vi "Periodic Tasks.vi"(8 "error in":errorcluster) -> ()   [LabVIEW 2013]
doc: "This VI runs in parallel to other tasks. It can contain as many user-defined periodic loops as you need. These can carry out PID or other sorts of timed response."
uses:
  <vilib>/Rock Robotics/SystemInterfaces/Utilities/FPGA_UtilitiesLED Source.ctl
  <vilib>/Rock Robotics/SystemInterfaces/Utilities/FPGA_UtilitiesLED State.ctl
  Robot Global Data.vi
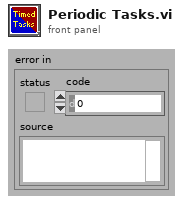
[diagram p1: front panel]
types:
  T1 = typedef "FPGA_UtilitiesLED State.ctl" = enum16{"Off", "On", "Toggle"}
  T2 = typedef "FPGA_UtilitiesLED Source.ctl" = enum16{"User LED", "FPGA LED"}
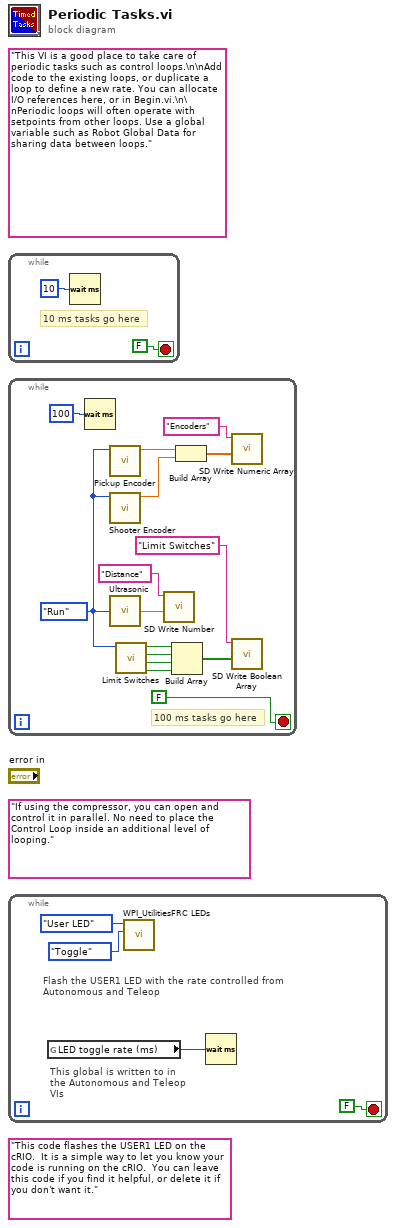
[diagram p0: block diagram]
diagram:
  (unwired) "If using the compressor, you can open and control it in parallel. No need to place the Control Loop inside an additional level of looping."
  (unwired) "This code flashes the USER1 LED on the cRIO.  It is a simple way to let you know your code is running on the cRIO.  You can leave this code if you find it helpful, or delete it if you don't want it."
  (unwired) "This VI is a good place to take care of periodic tasks such as control loops.\n\nAdd code to the existing loops, or duplicate a loop to define a new rate. You can allocate I/O references here, or in Begin.vi.\n\nPeriodic loops will often operate with setpoints from other loops. Use a global variable such as Robot Global Data for sharing data between loops."
  n1 = while {
    stop <- FALSE stop-if-true
    # "10 ms tasks go here"
    n2 = Wait (ms)(milliseconds to wait=u32 10) -> ()  [unwired: 1 out]
  }
  n3 = while {
    stop <- FALSE stop-if-true
    w9 = enum16{"Open", "Run", "End"}."Run" ("State Control")
    # "100 ms tasks go here"
    n4 = Wait (ms)(milliseconds to wait=u32 100) -> ()  [unwired: 1 out]
    n5 = call "Pickup Encoder.vi"("State Control"=w9) -> ("Encoder Degrees"=w8:dbl)  [unwired: 3 in, 3 out]
    n6 = call "Shooter Encoder.vi"("State Control"=w9) -> ("Encoder Degrees"=w7:dbl)  [unwired: 3 in, 3 out]
    n7 = call "Ultrasonic.vi"("State Control"=w9) -> ("Distance (in.)"=w4:dbl)
    n8 = call "Limit Switches.vi"("State Control"=w9) -> ("Shooter Top"=w10:bool, "Shooter Bottom"=w11:bool, "Picker Upper Bottom"=w12:bool, "Picker Upper Top"=w13:bool)  [unwired: 7 in]
    n9 = call <vilib>:"SD Write Number.vi"("Numeric"=w4, "Name"="Distance") -> ()  [unwired: 8 in, 2 out]
    n10 = Build Array(w13, w12, w11, w10) -> (w15:bool[])
    n11 = Build Array(w8, w7) -> (w6:dbl[])
    n12 = call <vilib>:"SD Write Numeric Array.vi"("Numeric Array"=w6, "Name"="Encoders") -> ()  [unwired: 8 in, 2 out]
    n13 = call <vilib>:"SD Write Boolean Array.vi"("Boolean Array"=w15, "Name"="Limit Switches") -> ()  [unwired: 8 in, 2 out]
  }
  n14 = while {
    stop <- FALSE stop-if-true
    # "This global is written to in the Autonomous and Teleop VIs"
    # "Flash the USER1 LED with the rate controlled from Autonomous and Teleop"
    n15 = global read "Robot Global Data.vi" "LED toggle rate (ms)"() -> (w18:u32)
    n16 = call <vilib>:"WPI_UtilitiesFRC LEDs.vi"("State"=FPGA_UtilitiesLED_State."Toggle", "LED Type"=FPGA_UtilitiesLED_Source."User LED") -> ()  [unwired: 1 in, 9 out]
    n17 = Wait (ms)(milliseconds to wait=w18) -> ()  [unwired: 1 out]
  }
